vi "UsrProfiles-Bundle changed params info.vi"(9 "Current value":dbl, 10 "Saved value":dbl, 11 "Cluster in":T1) -> (3 "Cluster out":T2)   [LabVIEW 2020]
uses:
  Typedefs/Changed parameter cluster.ctl
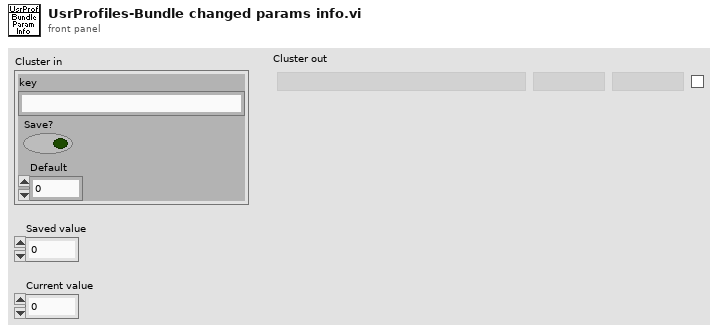
[diagram p1: front panel]
types:
  T1 = cluster{"key":string, "Save?":bool, "Default":dbl}
  T2 = typedef "Changed parameter cluster.ctl" = cluster{"Name":string, "Old value":string, "New value":string, "Save":bool}
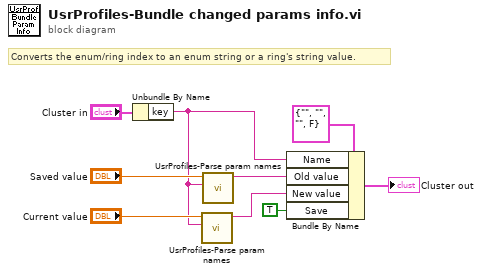
[diagram p0: block diagram]
diagram:
  # "Converts the enum/ring index to an enum string or a ring's string value."
  n1 = Unbundle By Name("Cluster in") -> ("key"=w1:string)
  n2 = call "UsrProfiles-Parse param names.vi"("key"=w1, "Saved value"="Current value") -> ("String"=w5:string)  [unwired: 9 in]
  n3 = call "UsrProfiles-Parse param names.vi"("key"=w1, "Saved value"="Saved value") -> ("String"=w4:string)  [unwired: 9 in]
  n4 = Bundle By Name(cluster=T2 {"Name"="", "Old value"="", "New value"="", "Save"=FALSE} ("Cluster"), "Name"=w1, "Old value"=w4, "New value"=w5, "Save"=TRUE) -> (→"Cluster out":T2)
